vi "Filter.vi"(0 "data":waveform(dbl)) -> (1 "Dynamic Data":dynamicdata(waveform), 2 "FFT - (RMS)":dynamicdata(waveform))   [LabVIEW 2020]
uses:
  <vilib>/express/express analysis/Spectral/Block/exnSpectralBlock spectral measurements RMS poly.vi
  <vilib>/express/express analysis/Spectral/Block/exnSpectralBlock spectral measurements RMS DDT.vi
  <vilib>/express/express analysis/Spectral/XNode/ExpressSpectralMeasurementsBlockNode.xnode
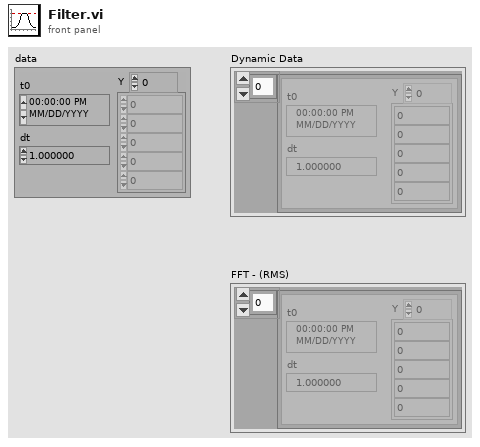
[diagram p1: front panel]
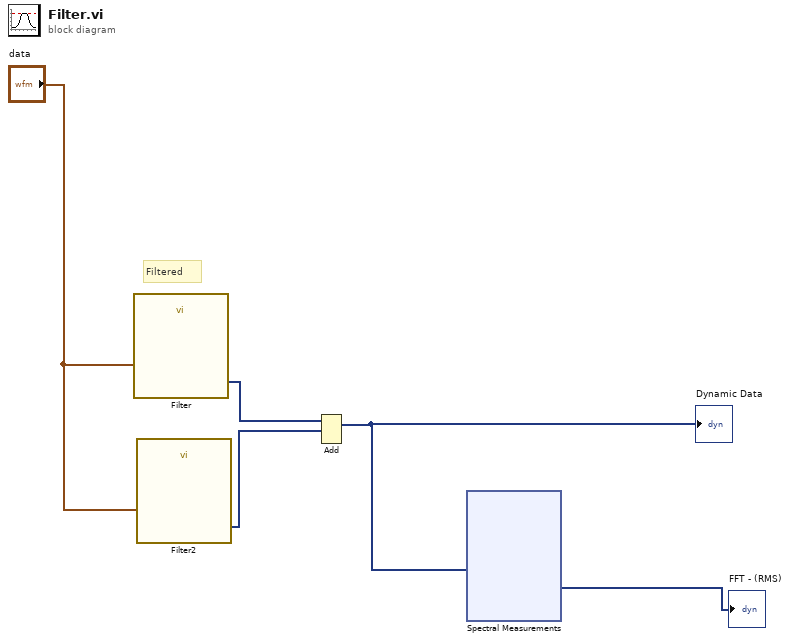
[diagram p0: block diagram]
diagram:
  # "Filtered"
  n1 = call "Filter"("Signal"="data") -> ("Filtered Signal"=w2:dynamicdata)  [unwired: 9 in, 1 out]
  n2 = call "Filter2"("Signal"="data") -> ("Filtered Signal"=w3:dynamicdata)  [unwired: 9 in, 1 out]
  n3 = Add(1:w3, 2:w2) -> (0:w5:dynamicdata)  [unwired: 1 in, 1 out]
  "Dynamic Data" <- w5
  n4 = xnode "Spectral Measurements"("Signals"=w5) -> ("FFT - (RMS)"=→"FFT - (RMS)":dynamicdata)  [unwired: 1 in, 2 out]
